vi "AddTaskIfCan.vi"   [LabVIEW 2012]
types:
  T1 = cluster{"Name":string, "Parameters":string[], "Start Conditional":cluster{"String":string, "avgs":cluster{"Expression":string, "Durration":dbl, "Replacement":string, "Values":dbl[]}[]}, "End Conditional":cluster{"String":string, "avgs":cluster{"Expression":string, "Durration":dbl, "Replacement":string, "Values":dbl[]}[]}, "Running":bool}[]
  T2 = cluster{"Name":string, "Parameters":string[], "Start Conditional":cluster{"String":string, "avgs":cluster{"Expression":string, "Durration":dbl, "Replacement":string, "Values":dbl[]}[]}, "End Conditional":cluster{"String":string, "avgs":cluster{"Expression":string, "Durration":dbl, "Replacement":string, "Values":dbl[]}[]}, "Running":bool}
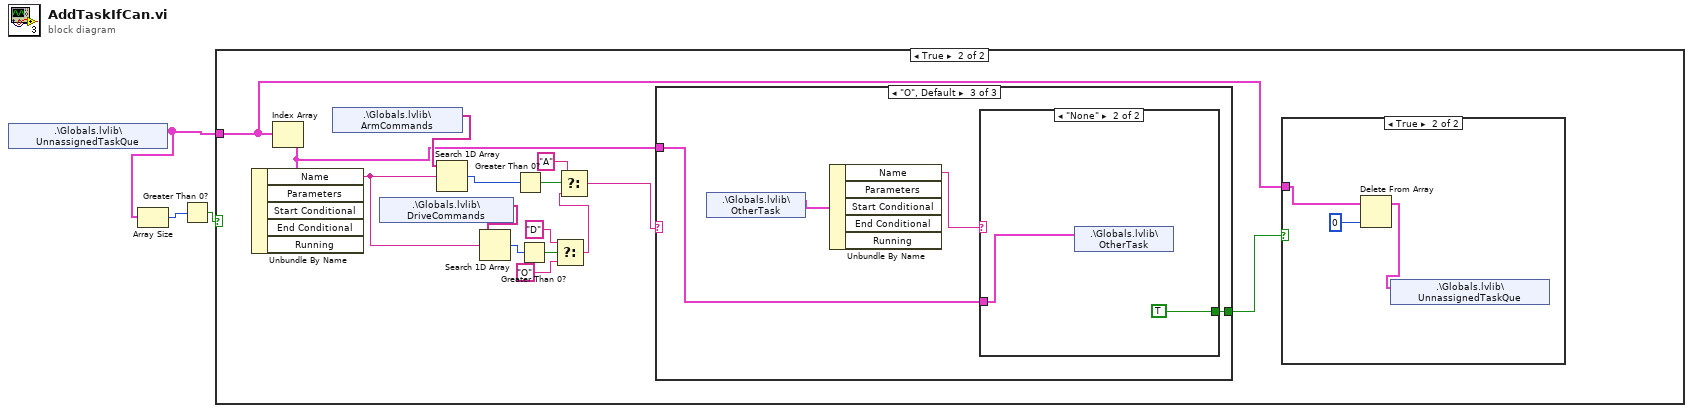
[diagram p0: block diagram]
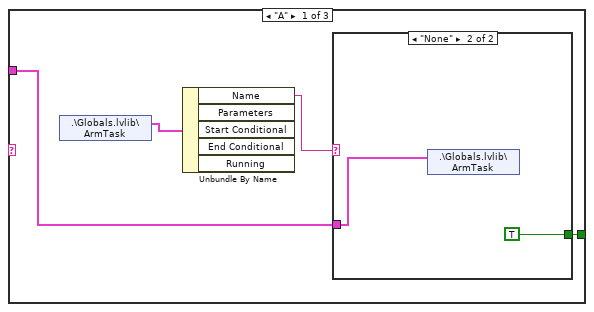
[diagram p4: hidden frame]
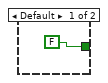
[diagram p5: hidden frame]
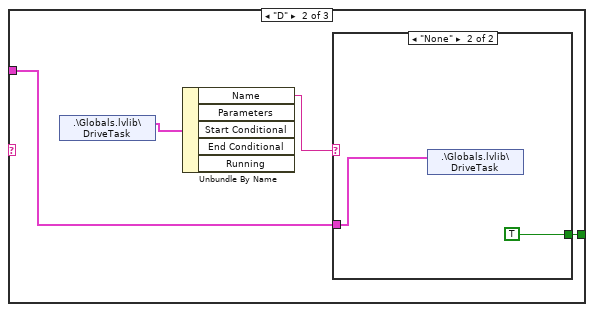
[diagram p6: hidden frame]
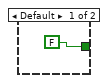
[diagram p7: hidden frame]
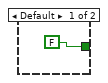
[diagram p8: hidden frame]
diagram:
  n1 = shared-variable ".\\Globals.lvlib\\UnnassignedTaskQue"() -> (w1:T1)  [unwired: 1 in, 1 out]
  n2 = Array Size(array=w1) -> (size(s)=w3:i32)
  n3 = Greater Than 0?(x=w3) -> (x > 0?=w2:bool)
  n4 = case shown="True" w2 {
    tunnel: w1 -> [_ w4]
    frame False {
    }
    frame True {
      n5 = Index Array(array=w4) -> (element=w6:T2)  [unwired: 1 in]
      n6 = Unbundle By Name(w6) -> ("Name"=w14:string)  [unwired: 4 out]
      n7 = shared-variable ".\\Globals.lvlib\\ArmCommands"() -> (w18:string[])  [unwired: 1 in, 1 out]
      n8 = shared-variable ".\\Globals.lvlib\\DriveCommands"() -> (w16:string[])  [unwired: 1 in, 1 out]
      n9 = Search 1D Array(1D array=w18, element=w14) -> (index of element=w17:i32)  [unwired: 1 in]
      n10 = Search 1D Array(1D array=w16, element=w14) -> (index of element=w15:i32)  [unwired: 1 in]
      n11 = Greater Than 0?(x=w17) -> (x > 0?=w8:bool)
      n12 = Greater Than 0?(x=w15) -> (x > 0?=w13:bool)
      n13 = Select(t="D", s=w13, f="O") -> (s? t:f=w9:string)
      n14 = Select(t="A", s=w8, f=w9) -> (s? t:f=w7:string)
      n15 = case shown="\"O\", Default" w7 {
        tunnel: w6 -> [w23 w30 w37]
        tunnel: [w22 w29 w36] -> w5
        frame "A" {
          n16 = shared-variable ".\\Globals.lvlib\\ArmTask"() -> (w25:T2)  [unwired: 1 in, 1 out]
          n17 = Unbundle By Name(w25) -> ("Name"=w24:string)  [unwired: 4 out]
          n18 = case shown="\"None\"" w24 {
            tunnel: w23 -> [_ w28]
            tunnel: [FALSE TRUE] -> w22
            frame Default {
            }
            frame "None" {
              n19 = shared-variable ".\\Globals.lvlib\\ArmTask"(w28) -> ()  [unwired: 1 in, 1 out]
            }
          }
        }
        frame "D" {
          n20 = shared-variable ".\\Globals.lvlib\\DriveTask"() -> (w32:T2)  [unwired: 1 in, 1 out]
          n21 = Unbundle By Name(w32) -> ("Name"=w31:string)  [unwired: 4 out]
          n22 = case shown="\"None\"" w31 {
            tunnel: w30 -> [_ w35]
            tunnel: [FALSE TRUE] -> w29
            frame Default {
            }
            frame "None" {
              n23 = shared-variable ".\\Globals.lvlib\\DriveTask"(w35) -> ()  [unwired: 1 in, 1 out]
            }
          }
        }
        frame "O", Default {
          n24 = shared-variable ".\\Globals.lvlib\\OtherTask"() -> (w39:T2)  [unwired: 1 in, 1 out]
          n25 = Unbundle By Name(w39) -> ("Name"=w38:string)  [unwired: 4 out]
          n26 = case shown="\"None\"" w38 {
            tunnel: w37 -> [_ w42]
            tunnel: [FALSE TRUE] -> w36
            frame Default {
            }
            frame "None" {
              n27 = shared-variable ".\\Globals.lvlib\\OtherTask"(w42) -> ()  [unwired: 1 in, 1 out]
            }
          }
        }
      }
      n28 = case shown="True" w5 {
        tunnel: w4 -> [_ w21]
        frame False {
        }
        frame True {
          n29 = Delete From Array(array=w21, index=0) -> (array with subset deleted=w19:T1)  [unwired: 1 in, 1 out]
          n30 = shared-variable ".\\Globals.lvlib\\UnnassignedTaskQue"(w19) -> ()  [unwired: 1 in, 1 out]
        }
      }
    }
  }
